vi "init.vi"(8 "error in (no error)":errorcluster, 10 "Device in":T1, 11 "data passing":T2) -> (0 "error out":errorcluster, 3 "data passing out":T2)   [LabVIEW 2016]
uses:
  data.ctl
  device.ctl
  <vilib>/Instr/_visa.llb/VISA Configure Serial Port (Instr).vi
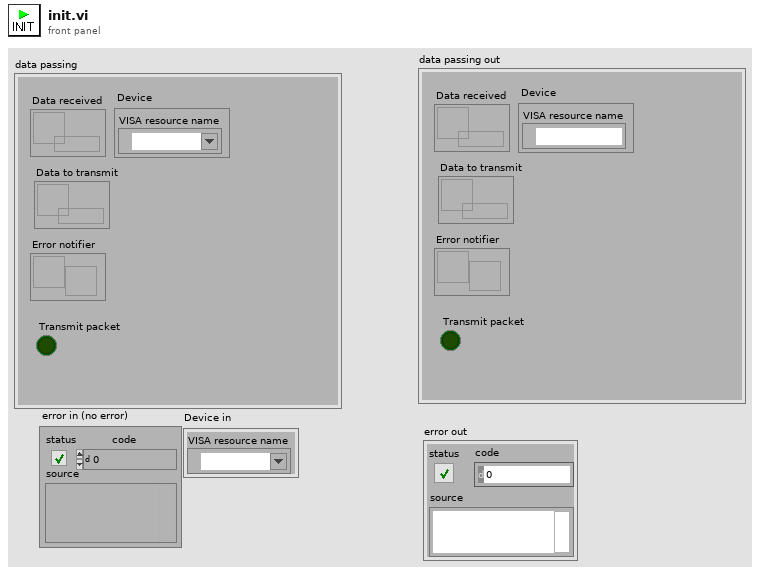
[diagram p1: front panel]
types:
  T1 = typedef "device.ctl" = cluster{"VISA resource name":refnum<visa-resource-name>}
  T2 = typedef "data.ctl" = cluster{"Data received":refnum<queue>, "Data to transmit":refnum<queue>, "Error notifier":refnum<notifier>, "Device":T1, "Transmit packet":bool}
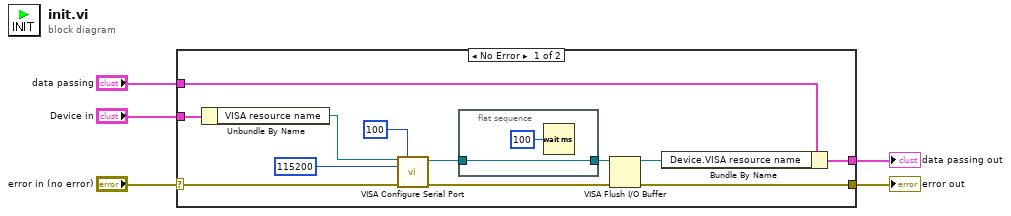
[diagram p0: block diagram]
diagram:
  n1 = case shown="No Error" "error in (no error)" {
    selector: "error in (no error)" -> [w17 w21]
    tunnel: [w6 w20] -> w2
    tunnel: "Device in" -> [w10 _]
    tunnel: [w16 w21] -> w1
    tunnel: "data passing" -> [w8 w20]
    frame No Error {
      n2 = Unbundle By Name(w10) -> ("VISA resource name"=w9:refnum<visa-resource-name>)
      n3 = call-poly "VISA Configure Serial Port"("VISA resource name"=w9, "timeout (10sec)"=u32 100, "baud rate (9600)"=u32 115200, "error in (no error)"=w17) -> ("VISA resource name out"=w12:refnum<visa-resource-name>, "error out"=w15:errorcluster)  [unwired: 5 in, 5 out]
      n4 = flat-sequence {
        tunnel: [w19] -> w13
        tunnel: w12 -> [w19]
        frame #0 {
          n5 = Wait (ms)(milliseconds to wait=u32 100) -> ()  [unwired: 1 out]
        }
      }
      n6 = VISA Flush I/O Buffer(VISA resource name=w13, error in (no error)=w15) -> (VISA resource name out=w7:refnum<visa-resource-name>, error out=w16:errorcluster)  [unwired: 1 in]
      n7 = Bundle By Name(cluster=w8, "Device.VISA resource name"=w7) -> (w6:T2)
    }
    frame Error {
    }
  }
  "data passing out" <- w2
  "error out" <- w1
